vi "Configure Wavelength Calibration Coefficient.vi"(6 "3rd Order Wavelength Calibration Coefficient":dbl format="%#_15g", 7 "0th Order Wavelength Calibration Coefficient":dbl format="%#_15g", 8 "error in (no error)":errorcluster, 9 "2nd Order Wavelength Calibration Coefficient":dbl format="%#_15g", 10 "1st Order Wavelength Calibration Coefficient":dbl format="%#_15g", 11 "VISA resource name":refnum<visa-resource-name>) -> (0 "error out":errorcluster, 3 "VISA resource name out":refnum<visa-resource-name>)   [LabVIEW 2021, in "Ocean Optics 2000 4000.lvlib"]
doc: "Configures the wavelength calibration coefficients. These coefficients will be saved in the EEPROM. \n\n<b>Note:</b>\nThis VI is reserved for advanced users. Changing these values may cause the spectrometer to be wrongly calibrated.\nConsult support from Ocean Optics before running this VI!"
uses:
  <instrlib>/Ocean Optics 2000 4000/Ocean Optics 2000 4000.lvlib
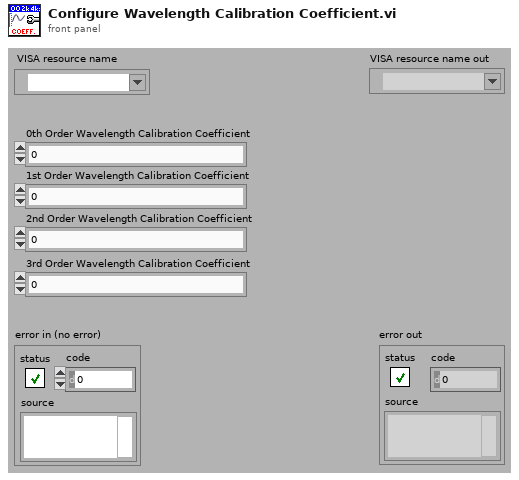
[diagram p1: front panel]
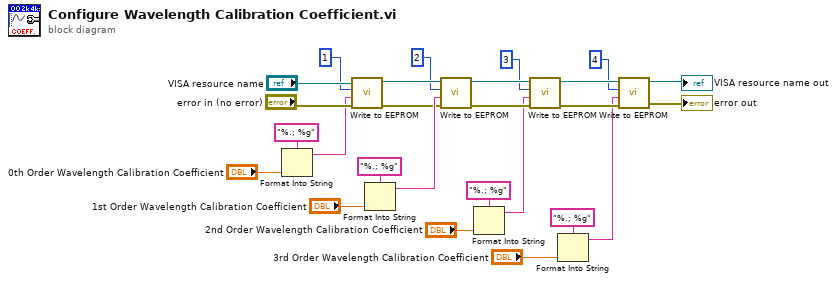
[diagram p0: block diagram]
diagram:
  n1 = Format Into String(format string="%.; %g", "0th Order Wavelength Calibration Coefficient") -> (resulting string=w21:string)  [unwired: 2 in, 1 out]
  n2 = call <instrlib>:"Write to EEPROM.vi"("error in (no error)"="error in (no error)", "15 Byte ASCII"=w21, "EEPROM Index"=u8 1, "VISA resource name"="VISA resource name") -> ("error out"=w14:errorcluster, "VISA resource name out"=w13:refnum<visa-resource-name>)  [unwired: 6 out]
  n3 = Format Into String(format string="%.; %g", "1st Order Wavelength Calibration Coefficient") -> (resulting string=w15:string)  [unwired: 2 in, 1 out]
  n4 = call <instrlib>:"Write to EEPROM.vi"("error in (no error)"=w14, "15 Byte ASCII"=w15, "EEPROM Index"=u8 2, "VISA resource name"=w13) -> ("error out"=w11:errorcluster, "VISA resource name out"=w12:refnum<visa-resource-name>)  [unwired: 6 out]
  n5 = Format Into String(format string="%.; %g", "2nd Order Wavelength Calibration Coefficient") -> (resulting string=w8:string)  [unwired: 2 in, 1 out]
  n6 = call <instrlib>:"Write to EEPROM.vi"("error in (no error)"=w11, "15 Byte ASCII"=w8, "EEPROM Index"=u8 3, "VISA resource name"=w12) -> ("error out"=w9:errorcluster, "VISA resource name out"=w10:refnum<visa-resource-name>)  [unwired: 6 out]
  n7 = Format Into String(format string="%.; %g", "3rd Order Wavelength Calibration Coefficient") -> (resulting string=w6:string)  [unwired: 2 in, 1 out]
  n8 = call <instrlib>:"Write to EEPROM.vi"("error in (no error)"=w9, "15 Byte ASCII"=w6, "EEPROM Index"=u8 4, "VISA resource name"=w10) -> ("error out"=→"error out":errorcluster, "VISA resource name out"=→"VISA resource name out":refnum<visa-resource-name>)  [unwired: 6 out]
